vi "Destroy ACQ User Events.vi"(8 "error in (no error)":errorcluster, 11 "ACQ Contador in":refnum<class "ACQ Contador.lvclass">) -> (0 "error out":errorcluster, 3 "ACQ Contador out":refnum<class "ACQ Contador.lvclass">)   [LabVIEW 2020, in "ACQ Contador.lvlib" / "ACQ Contador.lvclass"]
uses:
  ACQ Contador.lvclass
  ACQ Contador.lvclass/ACQ Contador.ctl
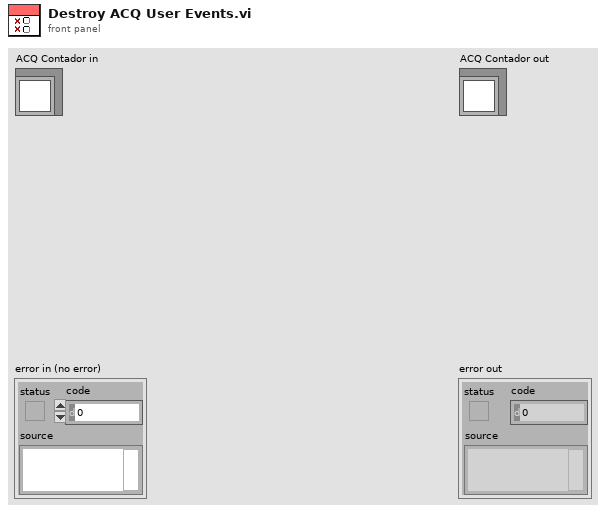
[diagram p1: front panel]
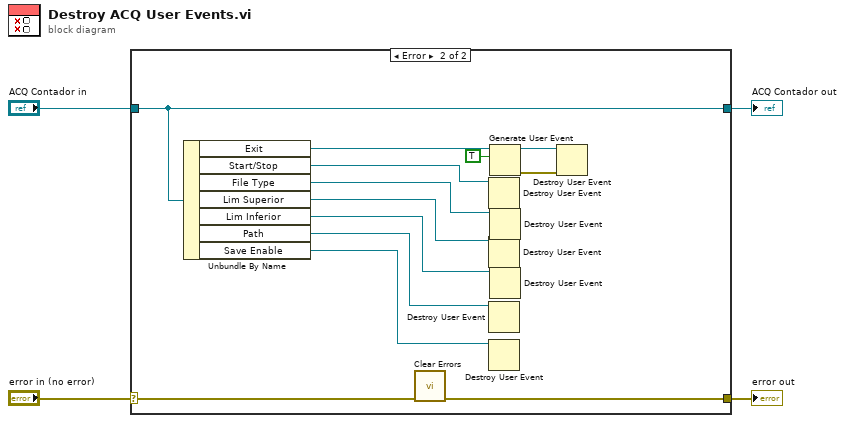
[diagram p0: block diagram]
diagram:
  n1 = case shown="Error" "error in (no error)" {
    selector: "error in (no error)" -> [w6 w19]
    tunnel: [w6 w7] -> w3
    tunnel: [w5 w18] -> w1
    tunnel: "ACQ Contador in" -> [w5 w18]
    frame No Error {
    }
    frame Error {
      n2 = Unbundle By Name(w18) -> ("Exit"=w17:refnum<user-event>, "Start/Stop"=w14:refnum<user-event>, "File Type"=w13:refnum<user-event>, "Lim Superior"=w12:refnum<user-event>, "Lim Inferior"=w11:refnum<user-event>, "Path"=w10:refnum<user-event>, "Save Enable"=w9:refnum<user-event>)
      n3 = call <vilib>:"Clear Errors.vi"("error in (no error)"=w19) -> ("error out"=w7:errorcluster)  [unwired: 5 in, 1 out]
      n4 = Destroy User Event(user event=w14) -> ()  [unwired: 1 in, 1 out]
      n5 = Destroy User Event(user event=w12) -> ()  [unwired: 1 in, 1 out]
      n6 = Destroy User Event(user event=w10) -> ()  [unwired: 1 in, 1 out]
      n7 = Destroy User Event(user event=w9) -> ()  [unwired: 1 in, 1 out]
      n8 = Generate User Event(user event=w17, event data cluster=TRUE ("event data")) -> (user event out=w16:refnum<user-event>, error out=w8:errorcluster)  [unwired: 2 in]
      n9 = Destroy User Event(user event=w13) -> ()  [unwired: 1 in, 1 out]
      n10 = Destroy User Event(user event=w11) -> ()  [unwired: 1 in, 1 out]
      n11 = Destroy User Event(user event=w16, error in=w8) -> ()  [unwired: 1 out]
    }
  }
  "error out" <- w3
  "ACQ Contador out" <- w1
